vi "oax_gs Load Data Sequence.vi"(9 "Select Data":string, 11 "value change":bool) -> (1 "load from daq file":bool, 2 "load tacho data":bool, 3 "load sv data":bool)   [LabVIEW 2017]
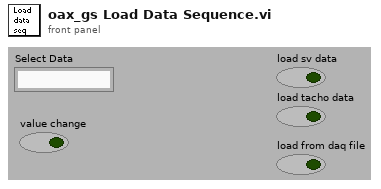
[diagram p1: front panel]
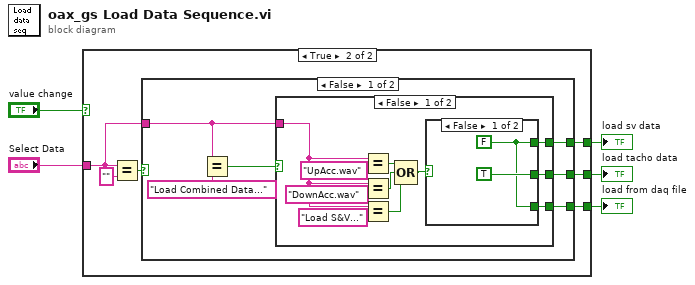
[diagram p0: block diagram]
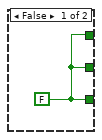
[diagram p2: hidden frame]
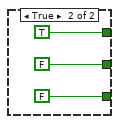
[diagram p3: hidden frame]
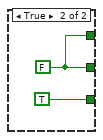
[diagram p4: hidden frame]
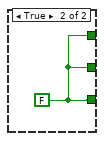
[diagram p5: hidden frame]
diagram:
  n1 = case shown="True" "value change" {
    tunnel: "Select Data" -> [_ w10]
    tunnel: [w6 w9] -> w3
    tunnel: [w6 w8] -> w2
    tunnel: [w6 w7] -> w1
    frame False {
      w6 = FALSE
    }
    frame True {
      n2 = Equal?(x=w10, y="") -> (x = y?=w11:bool)
      n3 = case shown="False" w11 {
        tunnel: w10 -> [w18 _]
        tunnel: [w15 w37] -> w9
        tunnel: [w14 w37] -> w8
        tunnel: [w13 w37] -> w7
        frame False {
          n4 = Equal?(x=w18, y="Load Combined Data...") -> (x = y?=w17:bool)
          n5 = case shown="False" w17 {
            tunnel: w18 -> [w21 _]
            tunnel: [w24 w35] -> w15
            tunnel: [w23 w35] -> w14
            tunnel: [w22 TRUE] -> w13
            frame False {
              n6 = Equal?(x=w21, y="UpAcc.wav") -> (x = y?=w27:bool)
              n7 = Equal?(x=w21, y="DownAcc.wav") -> (x = y?=w26:bool)
              n8 = Equal?(x=w21, y="Load S&V...") -> (x = y?=w19:bool)
              n9 = Compound Arithmetic op=OR(w27, w26, w19) -> (w25:bool)
              n10 = case shown="False" w25 {
                tunnel: [w30 TRUE] -> w24
                tunnel: [TRUE FALSE] -> w23
                tunnel: [w30 FALSE] -> w22
                frame False {
                  w30 = FALSE
                }
                frame True {
                }
              }
            }
            frame True {
              w35 = FALSE
            }
          }
        }
        frame True {
          w37 = FALSE
        }
      }
    }
  }
  "load sv data" <- w3
  "load tacho data" <- w2
  "load from daq file" <- w1
